vi "Read Result.vi"(8 "error in (no error)":errorcluster, 11 "Long Running Process in":refnum<class "Long Running Process.lvclass">) -> (0 "error out":errorcluster, 2 "Result":dbl, 3 "Long Running Process out":refnum<class "Long Running Process.lvclass">)   [LabVIEW 2017, in "Actor Example.lvlib" / "Long Running Process.lvclass"]
uses:
  Long Running Process.lvclass
  Long Running Process.lvclass/Long Running Process.ctl
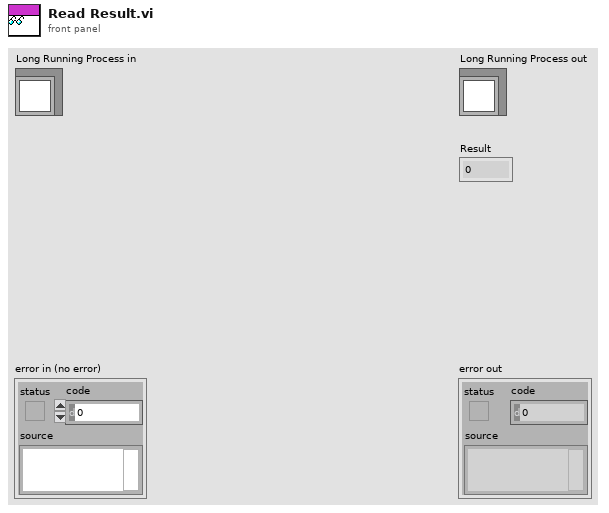
[diagram p1: front panel]
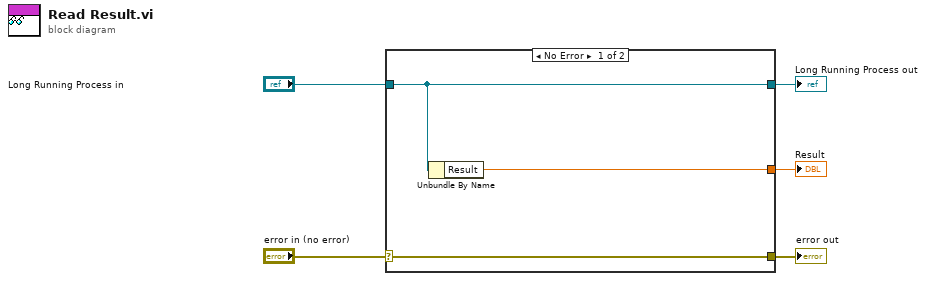
[diagram p0: block diagram]
diagram:
  n1 = case shown="No Error" "error in (no error)" {
    selector: "error in (no error)" -> [w8 w9]
    tunnel: [w8 w9] -> w4
    tunnel: [w7 w10] -> w2
    tunnel: "Long Running Process in" -> [w7 w10]
    tunnel: [w6 _] -> w1
    frame No Error {
      n2 = Unbundle By Name(w7) -> ("Result"=w6:dbl)
    }
    frame Error {
    }
  }
  "error out" <- w4
  "Long Running Process out" <- w2
  "Result" <- w1
